vi "HELP.vi"(8 "error in (no error)":errorcluster, 11 "Instrument in":refnum<class "Instrument.lvclass">) -> (0 "error out":errorcluster, 2 "Commands":string[](array[string]), 3 "Instrument in":refnum<class "Instrument.lvclass">)   [LabVIEW 2019, in "Instrument.lvclass"]
uses:
  Instrument.lvclass
  Typedefs/Instrument.Commands--Enum.ctl
  Instrument.lvclass/Instrument.ctl
  bb8a232c-f628-49fe-96b6-aa36c3f8e839.vi
  bb8a232c-f628-49fe-96b6-aa36c3f8e839.vi/cbbd5e4c-0643-493e-8b7e-2ac0e0644396.vi
  Send and Receive.vi
  bb8a232c-f628-49fe-96b6-aa36c3f8e839.vi/ad7a03f9-40d2-4f91-a86b-9df6fedd3f3b.vi
  Private/Get Client Type.vi
  bb8a232c-f628-49fe-96b6-aa36c3f8e839.vi/cbbd5e4c-0643-493e-8b7e-2ac0e0644396.vi/f88c764c-c3e3-46b7-b7e7-fa9ced24a985.vi
  bb8a232c-f628-49fe-96b6-aa36c3f8e839.vi/cbbd5e4c-0643-493e-8b7e-2ac0e0644396.vi/c0dd8680-f82c-409f-95f2-fe84c2776d0c.vi
  bb8a232c-f628-49fe-96b6-aa36c3f8e839.vi/ad7a03f9-40d2-4f91-a86b-9df6fedd3f3b.vi/77b1c17c-22df-46d0-9ad5-2d54c4a35d0e.vi
  bb8a232c-f628-49fe-96b6-aa36c3f8e839.vi/ad7a03f9-40d2-4f91-a86b-9df6fedd3f3b.vi/200e6d20-d191-40c8-a79b-8f2c3ce722e5.vi
  bb8a232c-f628-49fe-96b6-aa36c3f8e839.vi/ad7a03f9-40d2-4f91-a86b-9df6fedd3f3b.vi/77b1c17c-22df-46d0-9ad5-2d54c4a35d0e.vi/f6d6eb04-3ca9-4869-949f-11be4334beb1.vi
  bb8a232c-f628-49fe-96b6-aa36c3f8e839.vi/ad7a03f9-40d2-4f91-a86b-9df6fedd3f3b.vi/77b1c17c-22df-46d0-9ad5-2d54c4a35d0e.vi/12a96610-71c7-463d-80e6-9f6d400b34db.vi
  Private/Get RC Connection Status.vi
  Enum to String.vi
  <userlib>/LevyLab/RemoteControl/API/Send and Receive.vi
  <vilib>/Utility/Data Type/Get Type Information.vi
  <vilib>/JDP Science/JSONtext/JSON text to Variant.vi
  Instrument.GetPublicEvents.vi
  <vilib>/JDP Science/JSONtext/Variant to JSON Text.vi
  <vilib>/National Instruments/GUID Generator/Guid Generator.vi
  Instrument.MessageToProcess.vi
  Private/Instrument.MessageFromProcess.EventStructure.vi
  <vilib>/JDP Science/JSONtext/LVClass Serializer/JSONtext LVClass Serializer.lvclass
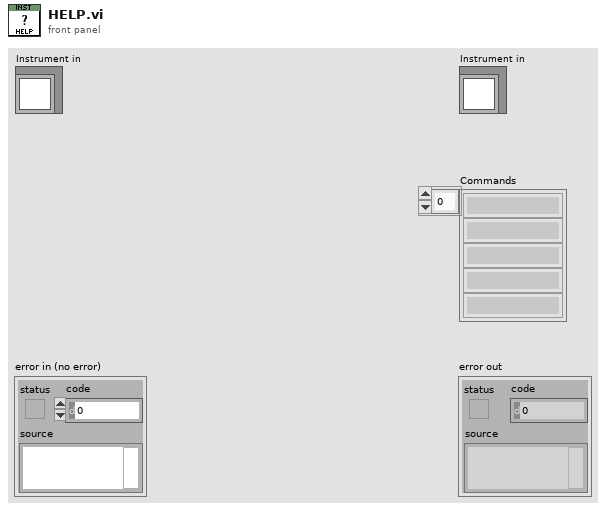
[diagram p1: front panel]
types:
  T1 = typedef "Instrument.lvclass/Instrument.Commands--Enum.ctl" = enum16{"HELP", "ACK", "setConfiguration", "getAll", "getAllData"}
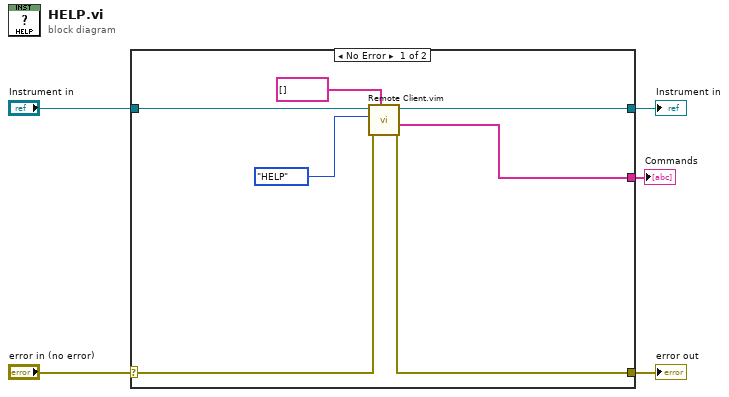
[diagram p0: block diagram]
diagram:
  n1 = case shown="No Error" "error in (no error)" {
    selector: "error in (no error)" -> [w10 w14]
    tunnel: [w7 w14] -> w4
    tunnel: [w12 w13] -> w2
    tunnel: "Instrument in" -> [w11 w13]
    tunnel: [w6 _] -> w1
    frame No Error {
      n2 = call "Remote Client.vim"("Data Out type"=string[] [] ("Commands"), "error in (no error)"=w10, "method"=Instrument.Commands--Enum."HELP" ("Commands"), "Instrument in"=w11) -> ("error out"=w7:errorcluster, "Data out"=w6:string[], "Instrument out"=w12:refnum<class "Instrument.lvclass">)  [unwired: 4 in, 1 out]
    }
    frame Error {
    }
  }
  "error out" <- w4
  "Instrument in" <- w2
  "Commands" <- w1
